vi "DMA Size Dist.vi"(4 "Selected Size":dbl, 5 "T":dbl, 6 "Qsample":dbl, 7 "Qaerosol":dbl, 8 "P":dbl, 9 "Qsheath":dbl, 10 "Qexcess":dbl, 11 "# of Charges":i32) -> (1 "V":dbl, 2 "Omega Function":T1, 3 "DMA Data Out":T2(array[cluster]))   [LabVIEW 2014]
uses:
  <vilib>/Analysis/1siggen.llb/Ramp Pattern by Samples.vi
  Atmospheric/Atmospheric Constants.vi
  DMA Constants.vi
  Conversion Constants.vi
  Atmospheric/Atmospheric Library.lvlib
  <vilib>/Analysis/NI_AALBase.lvlib
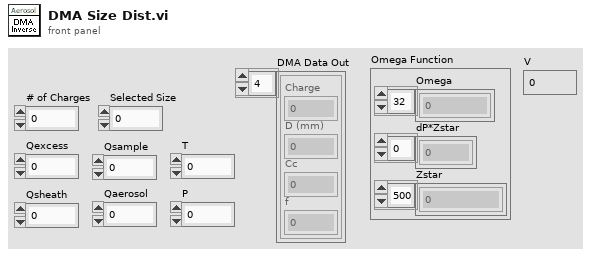
[diagram p1: front panel]
types:
  T1 = cluster{"Omega":dbl[], "dP*Zstar":dbl[], "Zstar":dbl[]}
  T2 = cluster{"Charge":i32, "D (mm)":dbl, "Cc":dbl, "f":dbl}[]
  T3 = cluster{"Charge":i32, "D (mm)":dbl, "Cc":dbl, "f":dbl}
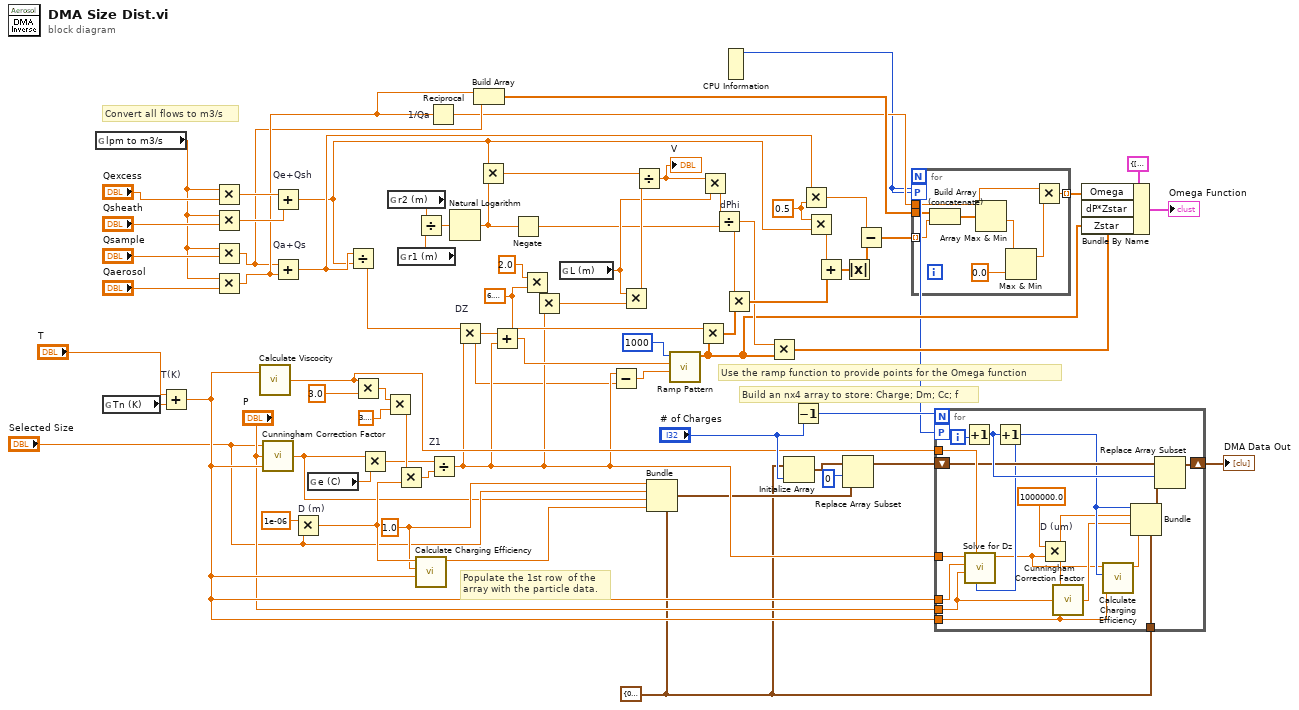
[diagram p0: block diagram]
diagram:
  w17 = T3 {"Charge"=0, "D (mm)"=0.0, "Cc"=0.0, "f"=0.0}
  w21 = 1.0 ("element")
  w22 = 0.5 ("y")
  w48 = 6.283185307179586
  # "Convert all flows to m3/s"
  # "Populate the 1st row  of the array with the particle data."
  # "Use the ramp function to provide points for the Omega function"
  # "Build an nx4 array to store: Charge; Dm; Cc; f"
  n1 = global read "Conversion Constants.vi" "lpm to m3/s"() -> (w68:dbl)
  n2 = global read "Atmospheric Constants.vi" "Tn (K)"() -> (w73:dbl)
  n3 = Add "T(K)"(x="T", y=w73) -> (x+y=w30:dbl)
  n4 = Multiply(x=w68, y="Qexcess") -> (x*y=w58:dbl)
  n5 = Multiply(x=w68, y="Qsheath") -> (x*y=w57:dbl)
  n6 = Multiply(x=w68, y="Qsample") -> (x*y=w40:dbl)
  n7 = Multiply(x=w68, y="Qaerosol") -> (x*y=w41:dbl)
  n8 = call "Calculate Viscocity.vi"("T(K)"=w30) -> ("mu (Pa*s)"=w31:dbl)  [unwired: 1 in]
  n9 = call "Cunningham Correction Factor.vi"("T (K)"=w30, "P (mb)"="P", "D (mm)"="Selected Size") -> ("Cc"=w15:dbl)
  n10 = Add "Qe+Qsh"(x=w58, y=w57) -> (x+y=w2:dbl)
  n11 = Add "Qa+Qs"(x=w40, y=w41) -> (x+y=w43:dbl)
  n12 = Multiply "D (m)"(x=1e-06, y="Selected Size") -> (x*y=w35:dbl)
  n13 = global read "Atmospheric Constants.vi" "e (C)"() -> (w67:dbl)
  n14 = Divide(x=w43, y=w2) -> (x/y=w53:dbl)
  n15 = Multiply(x=w31, y=3.0) -> (x*y=w65:dbl)
  n16 = Multiply(x=w15, y=w67) -> (x*y=w62:dbl)
  n17 = Multiply(x=w65, y=3.141592653589793) -> (x*y=w63:dbl)
  n18 = global read "DMA Constants.vi" "r2 (m)"() -> (w59:dbl)
  n19 = Multiply(x=w63, y=w35) -> (x*y=w61:dbl)
  n20 = global read "DMA Constants.vi" "r1 (m)"() -> (w60:dbl)
  n21 = Divide(x=w59, y=w60) -> (x/y=w7:dbl)
  n22 = call "Calculate Charging Efficiency.vi"("T (K)"=w30, "# of charges"=w21, "D (m)"=w35) -> ("f"=w19:dbl)  [unwired: 7 in, 1 out]
  n23 = Reciprocal "1/Qa"(x=w41) -> (1/x=w38:dbl)
  n24 = Divide "Z1"(x=w62, y=w61) -> (x/y=w26:dbl)
  n25 = Natural Logarithm(1:w7) -> (0:w5:dbl)
  n26 = Multiply "DZ"(x=w53, y=w26) -> (x*y=w25:dbl)
  n27 = Build Array(w41, w40) -> (w39:dbl[])
  n28 = Multiply(x=w2, y=w5) -> (x*y=w12:dbl)
  n29 = Add(x=w25, y=w26) -> (x+y=w50:dbl)
  n30 = Negate(x=w5) -> (-x=w6:dbl)
  n31 = Multiply(x=2.0, y=w48) -> (x*y=w56:dbl)
  n32 = Multiply(x=w56, y=w26) -> (x*y=w55:dbl)
  n33 = global read "DMA Constants.vi" "L (m)"() -> (w24:dbl)
  n34 = Subtract(x=w26, y=w25) -> (x-y=w51:dbl)
  n35 = Multiply(x=w24, y=w55) -> (x*y=w54:dbl)
  n36 = Divide ("V1")(x=w12, y=w54) -> (x/y=w23:dbl)
  "V" <- w23
  n37 = Bundle(cluster=w17, "Charge"=w21, "D (mm)"="Selected Size", "Cc"=w15, "f"=w19) -> (w18:T3)
  n38 = call-poly <vilib>:"Ramp Pattern.vi"("start"=w51, "end"=w50, "samples"=1000) -> ("Ramp Pattern"=w4:dbl[])  [unwired: 7 in, 1 out]
  n39 = Multiply(x=w48, y=w4) -> (x*y=w47:dbl[])
  n40 = Multiply(x=w23, y=w24) -> (x*y=w52:dbl)
  n41 = Divide "dPhi"(x=w52, y=w6) -> (x/y=w37:dbl)
  n42 = CPU Information() -> (4:w1:i32)  [unwired: 3 out]
  n43 = Multiply(x=w37, y=w47) -> (x*y=w46:dbl[])
  n44 = Multiply(x=w37, y=w4) -> (x*y=w11:dbl[])
  n45 = Initialize Array(w17, "# of Charges") -> (w36:T2)
  n46 = Decrement(x="# of Charges") -> (x-1=w32:i32)
  n47 = Multiply(x=w43, y=w22) -> (x*y=w42:dbl)
  n48 = Multiply(x=w22, y=w2) -> (x*y=w45:dbl)
  n49 = Add(x=w45, y=w46) -> (x+y=w44:dbl[])
  n50 = Replace Array Subset(array=w36, new element=w18, index=0 ("index (row)")) -> (w29:T2)
  n51 = Absolute Value(x=w44) -> (abs(x)=w9:dbl[])
  n52 = Subtract(x=w42, y=w9) -> (x-y=w10:dbl[])
  n53 = for {
    tunnel: w10 -> [w82] mode=indexing
    tunnel: w39 -> [w81]
    tunnel: w38 -> [w76]
    tunnel: [w75] -> w13 mode=indexing
    workers-P: w1 -> [_]
    n54 = Build Array (concatenate)(w81, w82) -> (w80:dbl[])
    n55 = Array Max & Min(array=w80) -> (min value=w79:dbl)  [unwired: 3 out]
    n56 = Max & Min(x=w79, y=0.0) -> (max(x,y)=w77:dbl)  [unwired: 1 out]
    n57 = Multiply(x=w76, y=w77) -> (x*y=w75:dbl)
  }
  n58 = for {
    N: w32 -> [_]
    tunnel: w26 -> [w98]
    tunnel: w30 -> [w97]
    tunnel: w31 -> [w96]
    tunnel: "P" -> [w91]
    tunnel: w30 -> [w95]
    shift-right: [w92] -> w16
    shift-left: w29 -> [w93]
    tunnel: w17 -> [w88]
    workers-P: w1 -> [_]
    i -> [w99]
    n59 = Increment(x=w99) -> (x+1=w94:i32)
    n60 = Increment(x=w94) -> (x+1=w89:i32)
    n61 = call "Solve for Dz.vi"("n"=w89, "mu"=w96, "P"=w91, "T"=w97, "Z1"=w98) -> ("dz"=w83:dbl)  [unwired: 5 in, 1 out]
    n62 = Multiply "D (um)"(x=1000000.0 ("y"), y=w83) -> (x*y=w87:dbl)
    n63 = call "Cunningham Correction Factor.vi"("T (K)"=w95, "P (mb)"=w91, "D (mm)"=w87) -> ("Cc"=w86:dbl)
    n64 = call "Calculate Charging Efficiency.vi"("T (K)"=w95, "# of charges"=w89, "D (m)"=w83) -> ("f"=w85:dbl)  [unwired: 7 in, 1 out]
    n65 = Bundle(cluster=w88, "Charge"=w89, "D (mm)"=w87, "Cc"=w86, "f"=w85) -> (w84:T3)
    n66 = Replace Array Subset(array=w93, new element=w84, index=w94) -> (w92:T2)
  }
  "DMA Data Out" <- w16
  n67 = Bundle By Name(cluster=T1 {"Omega"=[], "dP*Zstar"=[], "Zstar"=[]}, "Omega"=w13, "dP*Zstar"=w11, "Zstar"=w4) -> (→"Omega Function":T1)
